vi "Fin_GlobalPath.vi"() -> ()   [LabVIEW 2015]
panel:
  in  "AthinaOutDataDir":path=path "/home/atlas/Micromegas/ProdData"
  in  "DBpath":path=path "/home/atlas/Micromegas/ProdData/dbtxtfiles"
  in  "RootMacroDir":path=path "/home/atlas/Micromegas/root_macro"
  in  "ViDir":path=path "/home/atlas/Micromegas/interface"
  in  "OutDataDir":path=path "/home/atlas/Micromegas/ProdData"
  in  "LogFilesDir":path=path "/home/atlas/Micromegas/ProdData/C_CCD"
  in  "BinDir":path=path "/home/atlas/Micromegas/bin"
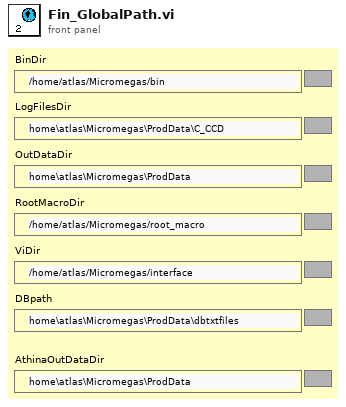
[diagram p1: front panel]
diagram:
